vi "HSV2RGB.vi"(3 "Value":dbl, 4 "Saturation":dbl, 5 "Hue":dbl) -> (0 "Blue":u8, 1 "Green":u8, 2 "Red":u8)   [LabVIEW 2013]
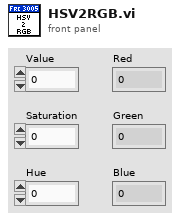
[diagram p1: front panel]
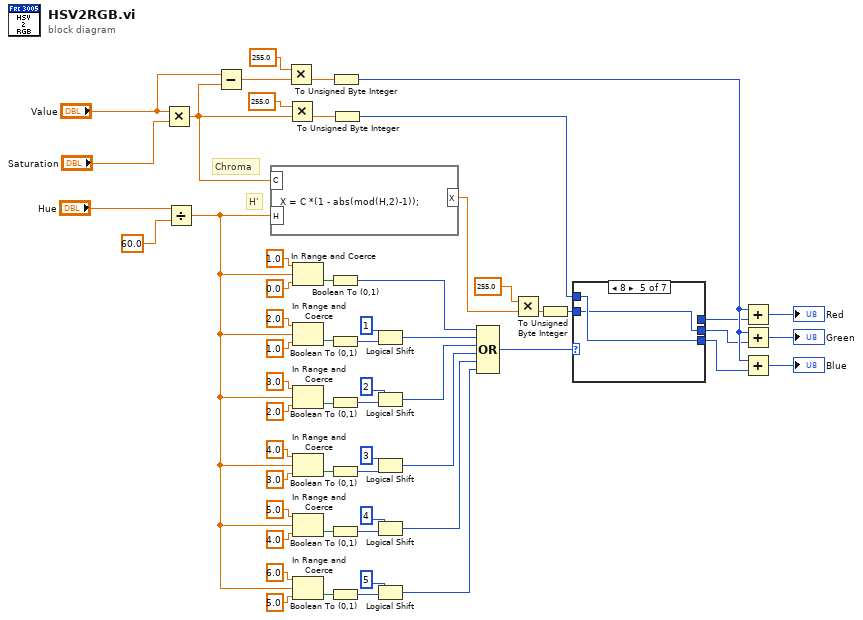
[diagram p0: block diagram]
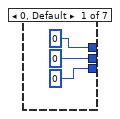
[diagram p2: hidden frame]
diagram:
  # "H'"
  # "Chroma"
  n1 = Multiply(x="Value", y="Saturation") -> (x*y=w26:dbl)
  n2 = Divide(x="Hue", y=60.0) -> (x/y=w16:dbl)
  n3 = Subtract(x="Value", y=w26) -> (x-y=w18:dbl)
  n4 = formula code="X = C *(1 - abs(mod(H,2)-1));"("C"=w26, "H"=w16) -> ("X"=w28:dbl)
  n5 = Multiply(x=255.0, y=w18) -> (x*y=w30:dbl)
  n6 = Multiply(x=255.0, y=w26) -> (x*y=w32:dbl)
  n7 = In Range and Coerce(upper limit=1.0, x=w16, lower limit=0.0) -> (In Range?=w37:bool)  [unwired: 1 out]
  n8 = In Range and Coerce(upper limit=2.0, x=w16, lower limit=1.0) -> (In Range?=w38:bool)  [unwired: 1 out]
  n9 = In Range and Coerce(upper limit=3.0, x=w16, lower limit=2.0) -> (In Range?=w39:bool)  [unwired: 1 out]
  n10 = In Range and Coerce(upper limit=4.0, x=w16, lower limit=3.0) -> (In Range?=w40:bool)  [unwired: 1 out]
  n11 = In Range and Coerce(upper limit=5.0, x=w16, lower limit=4.0) -> (In Range?=w41:bool)  [unwired: 1 out]
  n12 = In Range and Coerce(upper limit=6.0, x=w16, lower limit=5.0) -> (In Range?=w42:bool)  [unwired: 1 out]
  n13 = Boolean To (0,1)(Boolean=w37) -> (0, 1=w53:i16)
  n14 = Boolean To (0,1)(Boolean=w38) -> (0, 1=w43:i16)
  n15 = Boolean To (0,1)(Boolean=w39) -> (0, 1=w44:i16)
  n16 = Boolean To (0,1)(Boolean=w40) -> (0, 1=w45:i16)
  n17 = Boolean To (0,1)(Boolean=w41) -> (0, 1=w46:i16)
  n18 = Boolean To (0,1)(Boolean=w42) -> (0, 1=w47:i16)
  n19 = To Unsigned Byte Integer(number=w30) -> (unsigned 8bit integer=w23:u8)
  n20 = To Unsigned Byte Integer(number=w32) -> (unsigned 8bit integer=w27:u8)
  n21 = Logical Shift(y=i16 1, x=w43) -> (x << y=w52:i16)
  n22 = Logical Shift(y=i16 2, x=w44) -> (x << y=w51:i16)
  n23 = Logical Shift(y=i16 3, x=w45) -> (x << y=w50:i16)
  n24 = Logical Shift(y=i16 4, x=w46) -> (x << y=w49:i16)
  n25 = Logical Shift(y=i16 5, x=w47) -> (x << y=w48:i16)
  n26 = Compound Arithmetic op=OR(w53, w52, w51, w50, w49, w48) -> (w36:i16)
  n27 = Multiply(x=255.0, y=w28) -> (x*y=w34:dbl)
  n28 = To Unsigned Byte Integer(number=w34) -> (unsigned 8bit integer=w29:u8)
  n29 = case shown="8" w36 {
    tunnel: [u8 0 ("R") _ _ w66 w69 w70 w72] -> w24
    tunnel: [u8 0 ("R") w62 w65 w67 w68 _ _] -> w22
    tunnel: [u8 0 ("R") w63 w64 _ _ w71 w73] -> w19
    tunnel: w27 -> [_ w63 w65 w67 w69 w70 w73]
    tunnel: w29 -> [_ w62 w64 w66 w68 w71 w72]
    frame 0, Default {
    }
    frame 1 {
    }
    frame 2 {
    }
    frame 4 {
    }
    frame 8 {
    }
    frame 16 {
    }
    frame 32 {
    }
  }
  n30 = Add(x=w23, y=w19) -> (x+y=→"Red":u8)
  n31 = Add(x=w23, y=w22) -> (x+y=→"Green":u8)
  n32 = Add(x=w23, y=w24) -> (x+y=→"Blue":u8)
